vi "1-x-invdist.vi"(8 "err in":errorcluster, 9 "F(x)":dbl, 11 "p_LN":T1 caption="p_POI") -> (0 "err out":errorcluster caption="err  out", 1 "F(x)":dbl, 2 "x":dbl, 3 "p_LN":T1 caption="p_POI")   [LabVIEW 2010, in "lv_02.lvlib"]
uses:
  lv_02.lvlib
  p_5E1_LN.ctl
  <vilib>/gmath/statdist.llb/Normal Inverse CDF.vi
  <vilib>/gmath/NI_Gmath.lvlib
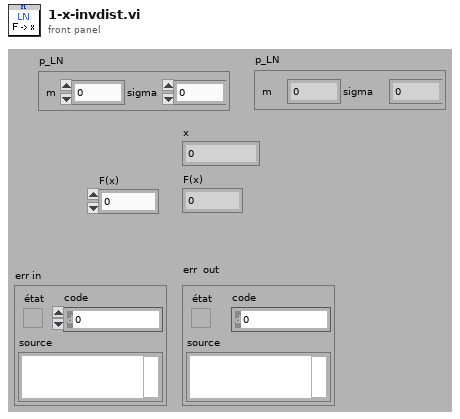
[diagram p1: front panel]
types:
  T1 = typedef "lv_02.lvlib/p_5E1_LN.ctl" = cluster{"m":dbl, "sigma":dbl}
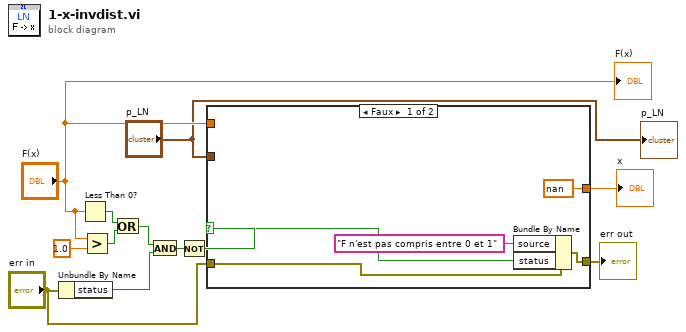
[diagram p0: block diagram]
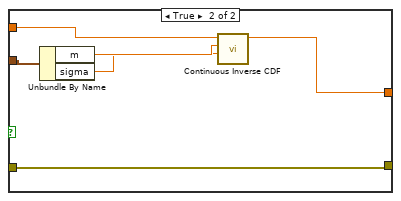
[diagram p2: hidden frame]
diagram:
  n1 = Unbundle By Name("err in") -> ("status"=w6:bool)
  n2 = Less Than 0?(x="F(x)") -> (x < 0?=w8:bool)
  n3 = Greater?(x="F(x)", y=1.0) -> (0:w9:bool)
  n4 = Or(x=w8, y=w9) -> (x .or. y?=w7:bool)
  n5 = And(x=w7, y=w6) -> (x .and. y?=w5:bool)
  n6 = Not(x=w5) -> (.not. x?=w4:bool)
  n7 = case shown="Faux" w4 {
    selector: w4 -> [w15 _]
    tunnel: "F(x)" -> [_ w20]
    tunnel: [nan ("x") w23] -> w12
    tunnel: "err in" -> [w16 w22]
    tunnel: [w17 w22] -> w2
    tunnel: "p_LN" -> [_ w21]
    frame False {
      n8 = Bundle By Name(cluster=w16, "source"="F n'est pas compris entre 0 et 1", "status"=w15) -> (w17:errorcluster)
    }
    frame True {
      n9 = Unbundle By Name(w21) -> ("m"=w19:dbl, "sigma"=w18:dbl)
      n10 = call-poly <vilib>:"Continuous Inverse CDF.vi"("std"=w18, "mean"=w19, "cdf(x)"=w20) -> ("x"=w23:dbl)  [unwired: 7 in, 1 out]
    }
  }
  "x" <- w12
  "err out" <- w2
  "F(x)" <- "F(x)"
  "p_LN" <- "p_LN"
